vi "LockinAux.vi"() -> ()   [LabVIEW 2013]
uses:
  <vilib>/Instr/_visa.llb/VISA Configure Serial Port (Instr).vi
panel:
  in  "1= -10 2=+10":bool
  in  "1= +10 2=-10":bool
  in  "Zero":bool
  in  "Both":bool
  in  "write2":bool
  in  "write1":bool
  out "Aux 2 Read":string="0\r"
  in  "Aux 2 Write":dbl=8.0
  in  "Step Time(s)":dbl=0.05
  in  "Step size(V)":dbl=0.025
  out "Aux 1 Read":string="0\r"
  in  "Aux 1 Write":dbl=-8.0
  in  "delay before read (ms)":u32=500
  in  "VISA resource name":refnum<visa-resource-name>="COM9"
  in  "stop":bool
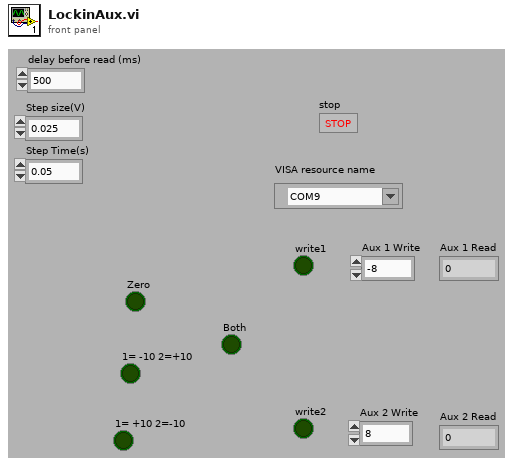
[diagram p1: front panel]
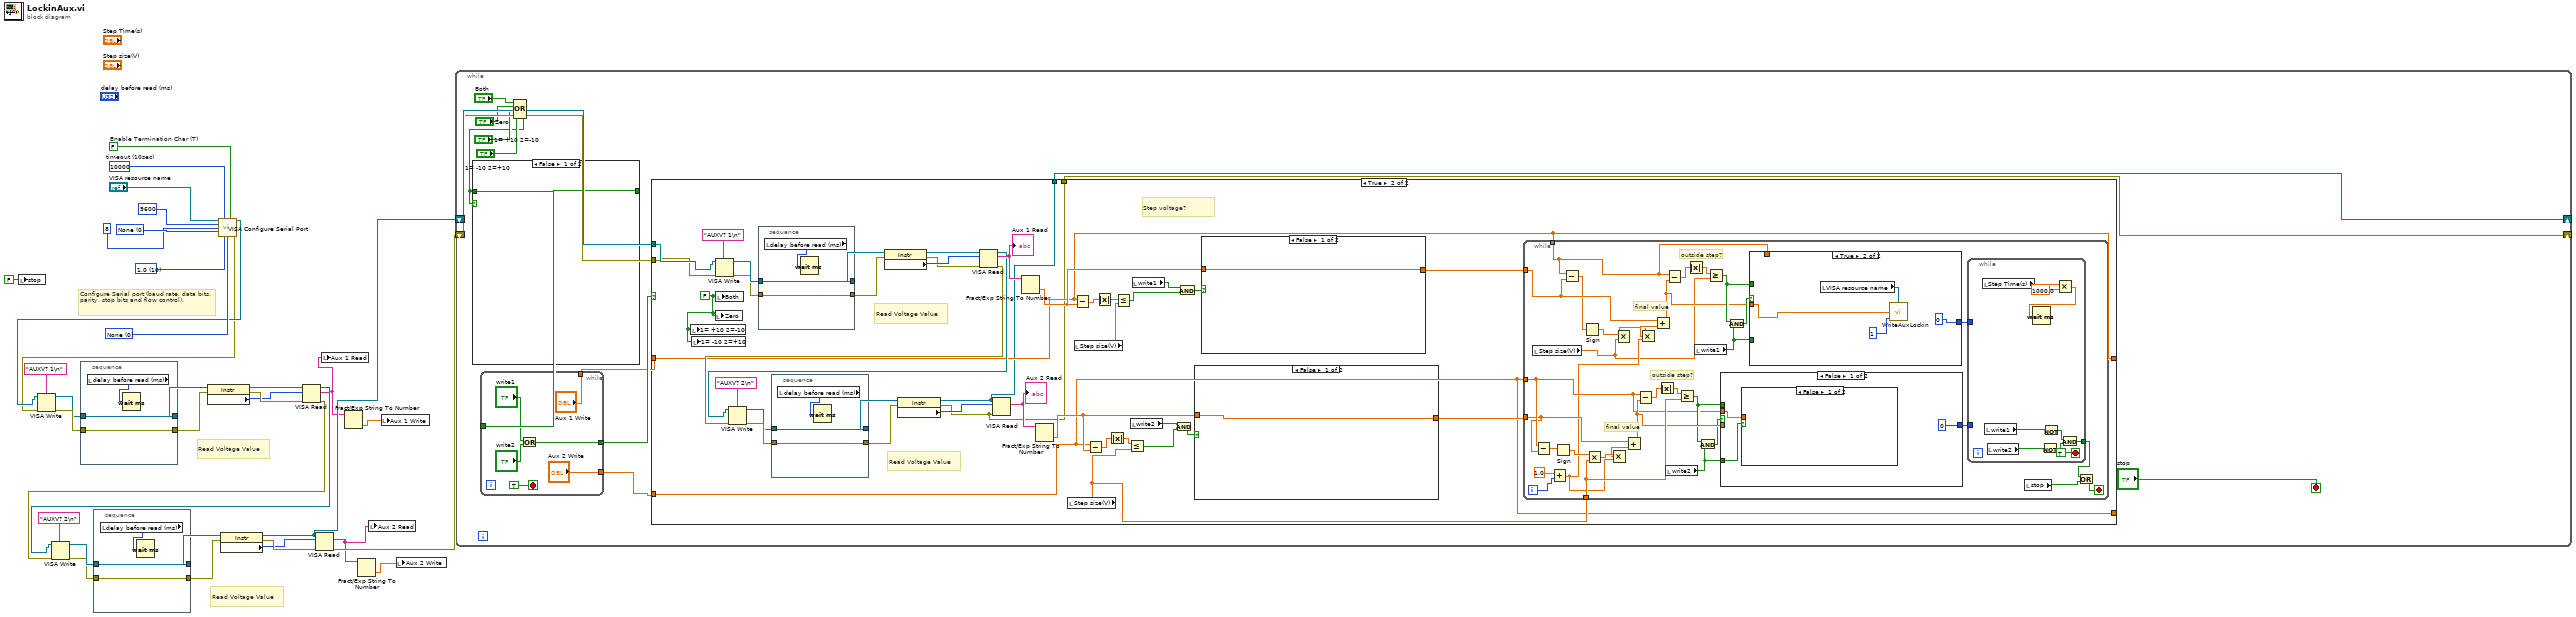
[diagram p0: block diagram]
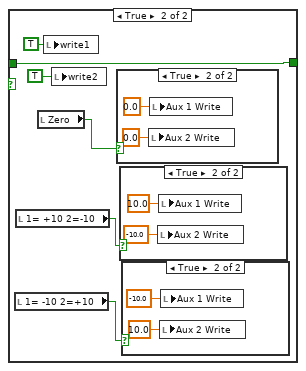
[diagram p2: hidden frame]
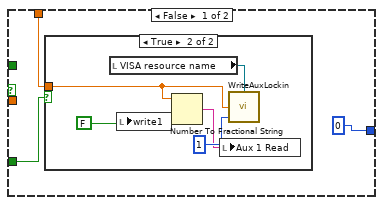
[diagram p7: hidden frame]
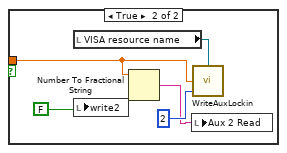
[diagram p9: hidden frame]
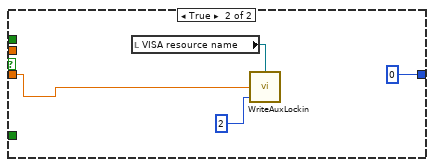
[diagram p10: hidden frame]
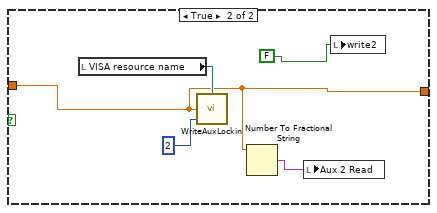
[diagram p11: hidden frame]
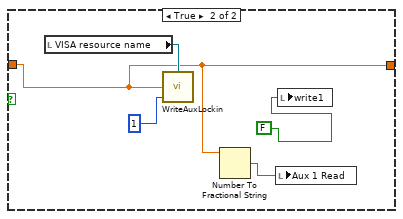
[diagram p12: hidden frame]
diagram:
  w28 = u16 0 items=["None"=0, "XON/XOFF"=1, "RTS/CTS"=2, "DTR/DSR"=4] ("flow control")
  w29 = u16 10 items=["1.0"=10, "1.5"=15, "2.0"=20] ("stop bits")
  w32 = u16 0 items=["None", "Odd", "Even", "Mark", "Space"] ("parity")
  w30 = FALSE  # Enable Termination Char (T)
  w31 = u32 10000  # timeout (10sec)
  # "Read Voltage Value"
  # "Read Voltage Value"
  # "Configure Serial port (baud rate, data bits, parity, stop bits and flow control)."
  n1 = local write "stop"(FALSE ("stop")) -> ()
  n2 = call-poly "VISA Configure Serial Port"("VISA resource name"="VISA resource name", "timeout (10sec)"=w31, "Enable Termination\nChar (T)"=w30, "baud rate (9600)"=u32 9600 ("baud rate"), "data bits (8)"=u16 8 ("data bits"), "parity (0:none)"=w32, "stop bits (10: 1 bit)"=w29, "flow control (0:none)"=w28) -> ("VISA resource name out"=w9:refnum<visa-resource-name>, "error out"=w8:errorcluster)  [unwired: 1 in, 5 out]
  n3 = VISA Write(VISA resource name=w9, write buffer="AUXV? 1\n" ("string to write"), error in (no error)=w8) -> (VISA resource name out=w15:refnum<visa-resource-name>, error out=w17:errorcluster)  [unwired: 1 out]
  n4 = stacked-sequence {
    tunnel: w17 -> [w37]
    tunnel: [w37] -> w16
    tunnel: w15 -> [w36]
    tunnel: [w36] -> w14
    frame #0 {
      n5 = local read "delay before read (ms)"() -> (w35:u32)
      n6 = Wait (ms)(milliseconds to wait=w35) -> ()  [unwired: 1 out]
    }
  }
  n7 = property class="Instr"(reference=w14, error in=w16) -> (reference out=w13:refnum<visa-resource-name>, error out=w12:errorcluster, "Serial Settings:Number of Bytes at Serial Port"=w11:u32)
  n8 = VISA Read(VISA resource name=w13, byte count=w11, error in (no error)=w12) -> (VISA resource name out=w25:refnum<visa-resource-name>, read buffer=w3:string, error out=w24:errorcluster)  [unwired: 1 out]
  n9 = VISA Write(VISA resource name=w25, write buffer="AUXV? 2\n" ("string to write"), error in (no error)=w24) -> (VISA resource name out=w20:refnum<visa-resource-name>, error out=w18:errorcluster)  [unwired: 1 out]
  n10 = stacked-sequence {
    tunnel: w18 -> [w40]
    tunnel: [w40] -> w19
    tunnel: w20 -> [w39]
    tunnel: [w39] -> w21
    frame #0 {
      n11 = local read "delay before read (ms)"() -> (w38:u32)
      n12 = Wait (ms)(milliseconds to wait=w38) -> ()  [unwired: 1 out]
    }
  }
  n13 = property class="Instr"(reference=w21, error in=w19) -> (reference out=w7:refnum<visa-resource-name>, error out=w26:errorcluster, "Serial Settings:Number of Bytes at Serial Port"=w22:u32)
  n14 = VISA Read(VISA resource name=w7, byte count=w22, error in (no error)=w26) -> (read buffer=w2:string, error out=w6:errorcluster)  [unwired: 2 out]
  n15 = local write "Aux 1 Read"(w3) -> ()
  n16 = Fract/Exp String To Number(string=w3) -> (number=w5:dbl)  [unwired: 3 in, 1 out]
  n17 = Fract/Exp String To Number(string=w2) -> (number=w4:dbl)  [unwired: 3 in, 1 out]
  n18 = local write "Aux 2 Read"(w2) -> ()
  n19 = local write "Aux 1 Write"(w5) -> ()
  n20 = local write "Aux 2 Write"(w4) -> ()
  n21 = while {
    shift-right: [w49] -> _
    shift-left: w7 -> [w53]
    shift-right: [w50] -> _
    shift-left: w6 -> [w52]
    stop <- "stop" stop-if-true
    n22 = Compound Arithmetic op=OR("Both", "Zero", "1= +10 2=-10", "1= -10 2=+10") -> (w41:bool)
    n23 = case shown="False" w41 {
      tunnel: [w55 w58] -> w48
      tunnel: w41 -> [w55 w58]
      frame False {
      }
      frame True {
        n24 = local read "1= -10 2=+10"() -> (w56:bool)
        n25 = local read "1= +10 2=-10"() -> (w57:bool)
        n26 = local read "Zero"() -> (w59:bool)
        n27 = local write "write1"(TRUE ("write1")) -> ()
        n28 = local write "write2"(TRUE ("write2")) -> ()
        n29 = case shown="True" w59 {
          frame False {
          }
          frame True {
            n30 = local write "Aux 2 Write"(0.0 ("Aux 2 Write")) -> ()
            n31 = local write "Aux 1 Write"(0.0 ("Aux 1 Write")) -> ()
          }
        }
        n32 = case shown="True" w57 {
          frame False {
          }
          frame True {
            n33 = local write "Aux 2 Write"(-10.0 ("Aux 2 Write")) -> ()
            n34 = local write "Aux 1 Write"(10.0 ("Aux 1 Write")) -> ()
          }
        }
        n35 = case shown="True" w56 {
          frame False {
          }
          frame True {
            n36 = local write "Aux 2 Write"(10.0 ("Aux 2 Write")) -> ()
            n37 = local write "Aux 1 Write"(-10.0 ("Aux 1 Write")) -> ()
          }
        }
      }
    }
    n38 = while {
      tunnel: [w73] -> w51
      tunnel: w48 -> [_]
      tunnel: ["Aux 1 Write"] -> w47
      tunnel: ["Aux 2 Write"] -> w46
      stop <- TRUE stop-if-true
      n39 = Or(x="write1", y="write2") -> (x .or. y?=w73:bool)
    }
    n40 = case shown="True" w51 {
      tunnel: w53 -> [w75 w110]
      tunnel: w52 -> [w74 w109]
      tunnel: w47 -> [w76 w82]
      tunnel: [w76 w82] -> _
      tunnel: w46 -> [w77 w81]
      tunnel: [w77 w81] -> _
      tunnel: [w75 w80] -> w49
      tunnel: [w74 w79] -> w50
      frame False {
      }
      frame True {
        w78 = FALSE ("Both")
        # "Read Voltage Value"
        # "Step voltage?"
        # "Read Voltage Value"
        n41 = local write "1= +10 2=-10"(w78) -> ()
        n42 = local write "1= -10 2=+10"(w78) -> ()
        n43 = VISA Write(VISA resource name=w110, write buffer="AUXV? 1\n" ("string to write"), error in (no error)=w109) -> (VISA resource name out=w113:refnum<visa-resource-name>, error out=w111:errorcluster)  [unwired: 1 out]
        n44 = local write "Zero"(w78) -> ()
        n45 = local write "Both"(w78) -> ()
        n46 = stacked-sequence {
          tunnel: w111 -> [w203]
          tunnel: [w203] -> w112
          tunnel: w113 -> [w202]
          tunnel: [w202] -> w114
          frame #0 {
            n47 = local read "delay before read (ms)"() -> (w201:u32)
            n48 = Wait (ms)(milliseconds to wait=w201) -> ()  [unwired: 1 out]
          }
        }
        n49 = property class="Instr"(reference=w114, error in=w112) -> (reference out=w115:refnum<visa-resource-name>, error out=w116:errorcluster, "Serial Settings:Number of Bytes at Serial Port"=w117:u32)
        n50 = VISA Read(VISA resource name=w115, byte count=w117, error in (no error)=w116) -> (VISA resource name out=w97:refnum<visa-resource-name>, read buffer=w108:string, error out=w98:errorcluster)  [unwired: 1 out]
        "Aux 1 Read" <- w108
        n51 = VISA Write(VISA resource name=w97, write buffer="AUXV? 2\n" ("string to write"), error in (no error)=w98) -> (VISA resource name out=w102:refnum<visa-resource-name>, error out=w104:errorcluster)  [unwired: 1 out]
        n52 = stacked-sequence {
          tunnel: w104 -> [w194]
          tunnel: [w194] -> w103
          tunnel: w102 -> [w193]
          tunnel: [w193] -> w101
          frame #0 {
            n53 = local read "delay before read (ms)"() -> (w192:u32)
            n54 = Wait (ms)(milliseconds to wait=w192) -> ()  [unwired: 1 out]
          }
        }
        n55 = property class="Instr"(reference=w101, error in=w103) -> (reference out=w80:refnum<visa-resource-name>, error out=w79:errorcluster, "Serial Settings:Number of Bytes at Serial Port"=w100:u32)
        n56 = VISA Read(VISA resource name=w80, byte count=w100, error in (no error)=w79) -> (read buffer=w105:string)  [unwired: 3 out]
        "Aux 2 Read" <- w105
        n57 = Fract/Exp String To Number(string=w108) -> (number=w106:dbl)  [unwired: 3 in, 1 out]
        n58 = Fract/Exp String To Number(string=w105) -> (number=w93:dbl)  [unwired: 3 in, 1 out]
        n59 = local read "Step size(V)"() -> (w94:dbl)
        n60 = Subtract(x=w82, y=w106) -> (x-y=w96:dbl)
        n61 = local read "Step size(V)"() -> (w107:dbl)
        n62 = Subtract(x=w81, y=w93) -> (x-y=w84:dbl)
        n63 = Absolute Value(x=w96) -> (abs(x)=w95:dbl)
        n64 = Absolute Value(x=w84) -> (abs(x)=w83:dbl)
        n65 = Less Or Equal?(x=w95, y=w107) -> (x <= y?=w86:bool)
        n66 = Less Or Equal?(x=w83, y=w94) -> (x <= y?=w89:bool)
        n67 = local read "write2"() -> (w90:bool)
        n68 = local read "write1"() -> (w87:bool)
        n69 = And(x=w90, y=w89) -> (x .and. y?=w88:bool)
        n70 = And(x=w87, y=w86) -> (x .and. y?=w85:bool)
        n71 = case shown="False" w88 {
          tunnel: w93 -> [w186 w188]
          tunnel: [w186 w188] -> w92
          frame False {
          }
          frame True {
            n72 = local read "VISA resource name"() -> (w191:refnum<visa-resource-name>)
            n73 = call "WriteAuxLockin.vi"("Output #"=2, "Voltage"=w188, "VISA resource name"=w191) -> ()
            n74 = Number To Fractional String(number=w188) -> (F-format string=w189:string)  [unwired: 3 in]
            n75 = local write "Aux 2 Read"(w189) -> ()
            n76 = local write "write2"(FALSE) -> ()
          }
        }
        n77 = case shown="False" w85 {
          tunnel: w106 -> [w195 w198]
          tunnel: [w195 w198] -> w91
          frame False {
          }
          frame True {
            n78 = local read "VISA resource name"() -> (w200:refnum<visa-resource-name>)
            n79 = call "WriteAuxLockin.vi"("Output #"=1, "Voltage"=w198, "VISA resource name"=w200) -> ()
            n80 = Number To Fractional String(number=w198) -> (F-format string=w197:string)  [unwired: 3 in]
            n81 = local write "Aux 1 Read"(w197) -> ()
            n82 = local write "write1"(FALSE) -> ()
          }
        }
        n83 = while {
          tunnel: w94 -> [w147]
          tunnel: w92 -> [w131]
          tunnel: w91 -> [w130]
          tunnel: w81 -> [w132]
          tunnel: w82 -> [w128]
          i -> [w126]
          stop <- w120 stop-if-true
          # "outside step?"
          # "final value"
          # "outside step?"
          # "final value"
          n84 = local read "Step size(V)"() -> (w124:dbl)
          n85 = Subtract(x=w132, y=w131) -> (x-y=w133:dbl)
          n86 = Add(x=1.0, y=w126) -> (x+y=w125:dbl)
          n87 = Sign(1:w133) -> (0:w152:dbl)
          n88 = Subtract(x=w128, y=w130) -> (x-y=w129:dbl)
          n89 = Sign(1:w129) -> (0:w134:dbl)
          n90 = Multiply(x=w152, y=w147) -> (x*y=w151:dbl)
          n91 = Multiply(x=w151, y=w125) -> (x*y=w150:dbl)
          n92 = Multiply(x=w134, y=w124) -> (x*y=w135:dbl)
          n93 = Add(x=w131, y=w150) -> (x+y=w146:dbl)
          n94 = Subtract(x=w132, y=w146) -> (x-y=w148:dbl)
          n95 = Multiply(x=w135, y=w125) -> (x*y=w136:dbl)
          n96 = Add(x=w130, y=w136) -> (x+y=w139:dbl)
          n97 = Absolute Value(x=w148) -> (abs(x)=w149:dbl)
          n98 = Subtract(x=w128, y=w139) -> (x-y=w138:dbl)
          n99 = local read "write2"() -> (w143:bool)
          n100 = Greater Or Equal?(x=w149, y=w147) -> (x >= y?=w144:bool)
          n101 = Absolute Value(x=w138) -> (abs(x)=w137:dbl)
          n102 = local read "write1"() -> (w142:bool)
          n103 = And(x=w144, y=w143) -> (x .and. y?=w145:bool)
          n104 = Greater Or Equal?(x=w137, y=w124) -> (x >= y?=w141:bool)
          n105 = case shown="False" w145 {
            tunnel: w146 -> [_ w185]
            tunnel: w144 -> [_ _]
            tunnel: w143 -> [w176 _]
            tunnel: w132 -> [w175 _]
            tunnel: [0 0] -> w122
            frame False {
              n106 = case shown="False" w176 {
                tunnel: w175 -> [_ w178]
                frame False {
                }
                frame True {
                  n107 = local read "VISA resource name"() -> (w181:refnum<visa-resource-name>)
                  n108 = local write "write2"(FALSE) -> ()
                  n109 = Number To Fractional String(number=w178) -> (F-format string=w177:string)  [unwired: 3 in]
                  n110 = local write "Aux 2 Read"(w177) -> ()
                  n111 = call "WriteAuxLockin.vi"("Output #"=2, "Voltage"=w178, "VISA resource name"=w181) -> ()
                }
              }
            }
            frame True {
              n112 = local read "VISA resource name"() -> (w182:refnum<visa-resource-name>)
              n113 = call "WriteAuxLockin.vi"("Output #"=2, "Voltage"=w185, "VISA resource name"=w182) -> ()
            }
          }
          n114 = And(x=w141, y=w142) -> (x .and. y?=w140:bool)
          n115 = case shown="True" w140 {
            tunnel: w139 -> [_ w173]
            tunnel: w141 -> [_ _]
            tunnel: w142 -> [w164 _]
            tunnel: w128 -> [w163 _]
            tunnel: [0 0] -> w123
            frame False {
              n116 = case shown="True" w164 {
                tunnel: w163 -> [_ w165]
                frame False {
                }
                frame True {
                  n117 = local read "VISA resource name"() -> (w169:refnum<visa-resource-name>)
                  n118 = local write "write1"(FALSE) -> ()
                  n119 = Number To Fractional String(number=w165) -> (F-format string=w166:string)  [unwired: 3 in]
                  n120 = local write "Aux 1 Read"(w166) -> ()
                  n121 = call "WriteAuxLockin.vi"("Output #"=1, "Voltage"=w165, "VISA resource name"=w169) -> ()
                }
              }
            }
            frame True {
              n122 = local read "VISA resource name"() -> (w170:refnum<visa-resource-name>)
              n123 = call "WriteAuxLockin.vi"("Output #"=1, "Voltage"=w173, "VISA resource name"=w170) -> ()
            }
          }
          n124 = while {
            tunnel: [w157] -> w121
            tunnel: w123 -> [_]
            tunnel: w122 -> [_]
            stop <- TRUE stop-if-true
            n125 = local read "Step Time(s)"() -> (w155:dbl)
            n126 = local read "write1"() -> (w161:bool)
            n127 = local read "write2"() -> (w160:bool)
            n128 = Not(x=w160) -> (.not. x?=w158:bool)
            n129 = Not(x=w161) -> (.not. x?=w159:bool)
            n130 = Multiply(x=w155, y=1000.0) -> (x*y=w154:dbl)
            n131 = Wait (ms)(milliseconds to wait=w154) -> ()  [unwired: 1 out]
            n132 = And(x=w159, y=w158) -> (x .and. y?=w157:bool)
          }
          n133 = local read "stop"() -> (w119:bool)
          n134 = Or(x=w121, y=w119) -> (x .or. y?=w120:bool)
        }
      }
    }
  }
